vi "AI-DO-DAQ-OneShot.vi"(6 "Signal Generation":T1={"Signal Type"=enum."Sine Wave", "Amplitude"=1.0, "frequency"=10.0} {"frequency" format="%0.2p"; "Amplitude" format="%0.2p"}, 7 "Timing Parameters":cluster{"Rate":dbl, "Length (s)":dbl}={"Rate"=10000.0, "Length (s)"=1000.0} {"Rate" format="%0.2f"}, 8 "error in (no error)":errorcluster, 10 "Output":T2={"Physical Channel"="Dev2/ai1", "Minimum Value"=-10.0, "Maximum Value"=10.0} {"Maximum Value" format="%0.2f"; "Minimum Value" format="%0.2f"}, 11 "Input":T2={"Physical Channel"="Dev2/ai1", "Minimum Value"=-10.0, "Maximum Value"=10.0} {"Maximum Value" format="%0.2f"; "Minimum Value" format="%0.2f"}) -> (0 "error out":errorcluster, 2 "Rate":dbl=10000.0 caption="Actual Rate" format="%0.2f", 3 "Measurement":waveform(dbl)(graph))   [LabVIEW 2014]
doc: "I. Description:\nThis example demonstrates how to continuously acquire and generate data at the same time, synchronized with one another.\n\nII. Instructions for Running:\n1. Select the physical channel to correspond to where your signal is input on the DAQ device. Also, select the corresponding channel for where your signal is being generated.\n2. Enter the minimum and maximum voltage ranges.\nNote: For better accuracy try to match the input range to the expected voltage level of the measured signal.\n3. Set the Input/Output rate of the acquisition.\nNote: The rate should be at least twice as fast as the maximum frequency component of the signal being acquired. \n4. Select what type of signal to generate and the amplitude.\nNote: This example requires two DMA channels to run. If your hardware does not support two DMA channels, you need to set the Data Transfer Mechanism property for the Analog Output Task to use \"Interrupts\". The Data Transfer Mechanism property is located in the DAQmx Channel Property hierarchy at:\n\nDAQmx Channel Property Node>>Analog Output>>General Properties>>Advanced>>Data Transfer and Memory>>Data Transfer Mechanism\n\nRefer to your device documentation to determine how many DMA channels are supported for your hardware.\n\nIII. Block Diagram Steps:\n1. Create an analog input voltage channel. Also, create an analog output voltage channel.\n2. Set the rate for the sample clock. Additionally, define the sample mode to be continuous. Also, set the sample clock rate for the signal generation.\n2a. Call the Get Terminal Name with Device Prefix VI. This will take a Task and a terminal and create a properly formatted device + terminal name to use as the source of analog output.\n3. Find out what our actual Input/Output rate is \n4. Use the Basic Function Generator VI to create the signal to be generated.\n5. Call the Start VI to arm the two functions. Make sure the analog output is armed before the analog input. This will ensure both will start at the same time.\n6. Read the waveform data in a loop until the user hits the stop button or an error occurs. The Is Task Done? VI is used to check for errors in the Analog Output Task.\n7. Call the Clear VI to Clear the Task\n8. Use the popup dialog box to display an error if any.\n\nIV. I/O Connections Overview:\nMake sure your signal input/output terminals match the Physical Channel I/O controls."
uses:
  <vilib>/DAQmx/create/channels.llb/DAQmx Create Channel (AO-Voltage-Basic).vi
  <vilib>/DAQmx/configure/timing.llb/DAQmx Timing (Sample Clock).vi
  <vilib>/DAQmx/write.llb/DAQmx Write (Analog Wfm 1Chan NSamp).vi
  <vilib>/DAQmx/create/channels.llb/DAQmx Create Channel (AI-Voltage-Basic).vi
  <vilib>/DAQmx/read.llb/DAQmx Read (Analog Wfm 1Chan NSamp).vi
  <vilib>/measure/NI_MABase.lvlib
  <resource>/objmgr/daqmx.rc
panel:
  # "Channel Parameters"
  # "Timing Parameters"
  # "Signal Generation"
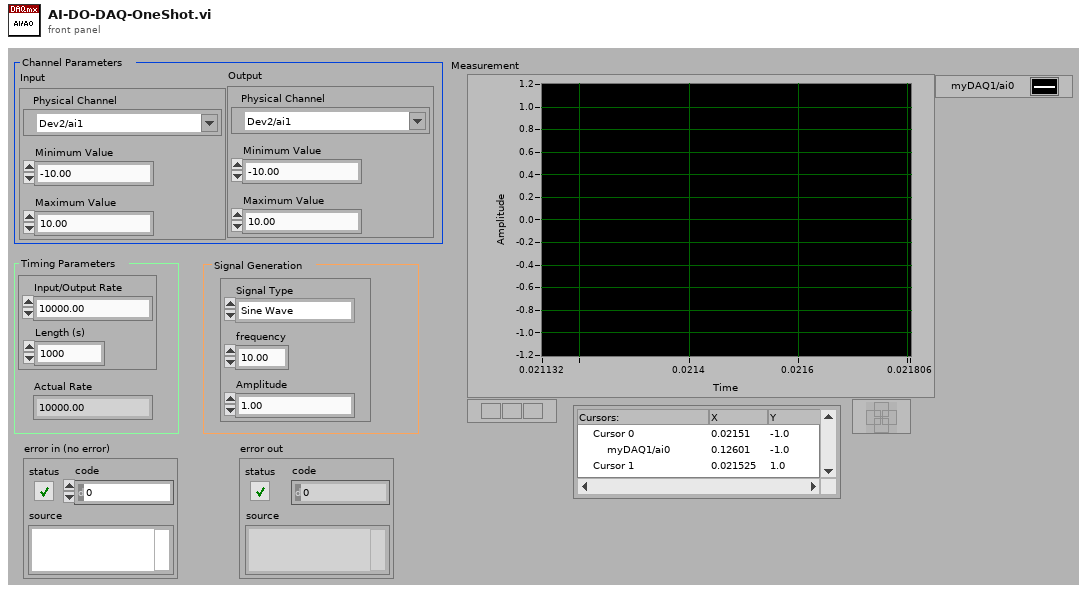
[diagram p1: front panel]
types:
  T1 = cluster{"Signal Type":enum16{"Sine Wave", "Triangle Wave", "Square Wave", "Sawtooth Wave"}, "Amplitude":dbl, "frequency":dbl}
  T2 = cluster{"Physical Channel":tag, "Minimum Value":dbl, "Maximum Value":dbl}
  T3 = enum16{"Sine Wave", "Triangle Wave", "Square Wave", "Sawtooth Wave"}
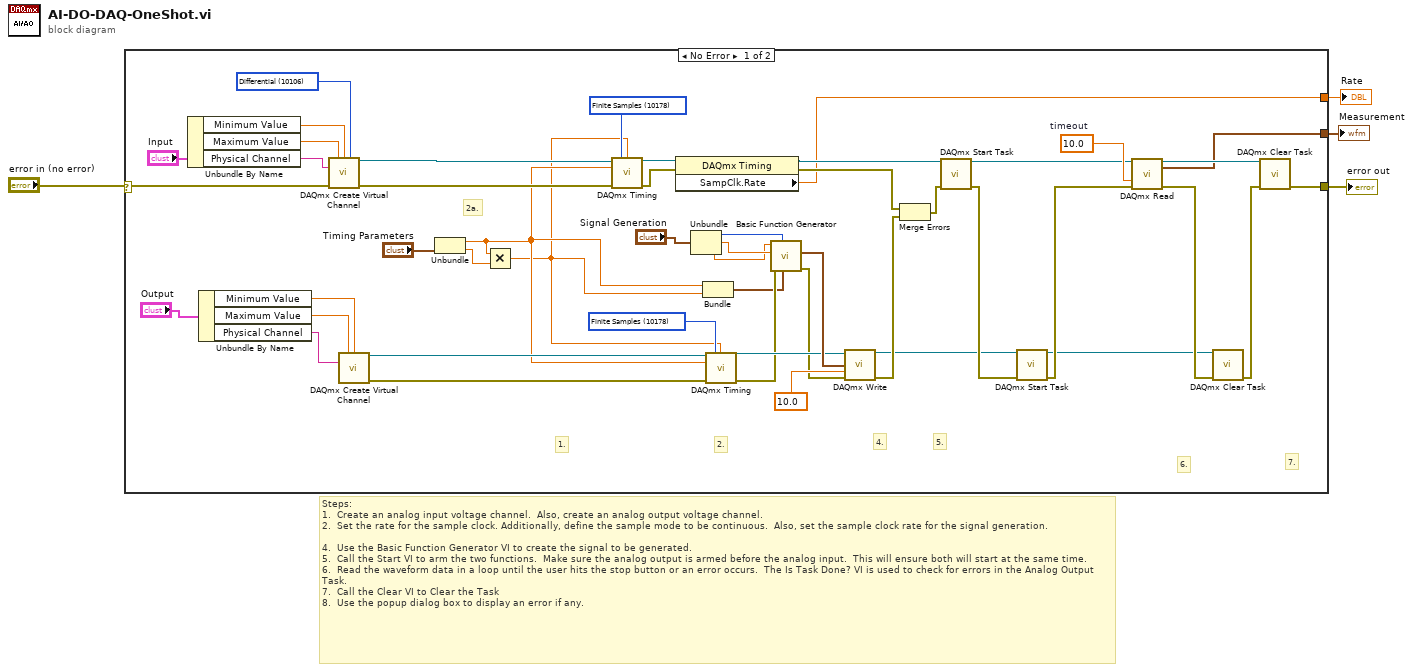
[diagram p0: block diagram]
diagram:
  # "Steps: \n1.  Create an analog input voltage channel.  Also, create an analog output voltage channel.\n2.  Set the rate for the sample clock. Additionally, define the sample mode to be continuous.  Also, set the sample clock rate for the signal generation.\n\n4.  Use the Basic Function Generator VI to create the signal to be generated.\n5.  Call the Start VI to arm the two functions.  Make sure the analog output is armed before the analog input.  This will ensure both will start at the same time.\n6.  Read the waveform data in a loop until the user hits the stop button or an error occurs.  The Is Task Done? VI is used to check for errors in the Analog Output Task.\n7.  Call the Clear VI to Clear the Task\n8.  Use the popup dialog box to display an error if any."
  n1 = case shown="No Error" "error in (no error)" {
    selector: "error in (no error)" -> [w10 w53]
    tunnel: [w44 w53] -> w3
    tunnel: [w9 _] -> w2
    tunnel: [w8 _] -> w1
    frame No Error {
      w31 = 10106 items=["default"=-1, "RSE"=10083, "NRSE"=10078, "Differential"=10106, "Pseudodifferential"=12529] ("input terminal configuration")
      w42 = 10.0  # timeout
      w50 = 10178 items=["Finite Samples"=10178, "Continuous Samples"=10123] ("sample mode")
      w51 = 10178 items=["Finite Samples"=10178, "Continuous Samples"=10123] ("sample mode")
      # "2a."
      # "6."
      # "4."
      # "5."
      # "7."
      # "2."
      # "1."
      n2 = Unbundle By Name("Input") -> ("Minimum Value"=w28:dbl, "Maximum Value"=w27:dbl, "Physical Channel"=w29:tag)
      n3 = Unbundle By Name("Output") -> ("Minimum Value"=w26:dbl, "Maximum Value"=w25:dbl, "Physical Channel"=w24:tag)
      n4 = call-poly <vilib>:"DAQmx Create Virtual Channel.vi"("maximum value"=w27, "minimum value"=w28, "input terminal configuration"=w31, "physical channels"=w29, "error in"=w10) -> ("task out"=w33:refnum<k21>, "error out"=w32:errorcluster)  [unwired: 9 in]
      n5 = call-poly <vilib>:"DAQmx Create Virtual Channel.vi"("maximum value"=w25, "minimum value"=w26, "physical channels"=w24) -> ("task out"=w49:refnum<k21>, "error out"=w48:errorcluster)  [unwired: 11 in]
      n6 = Unbundle("Timing Parameters") -> ("Rate"=w7:dbl, "Length (s)"=w11:dbl)
      n7 = Multiply(x=w7, y=w11) -> (x*y=w6:dbl)
      n8 = call-poly <vilib>:"DAQmx Timing.vi"("task/channels in"=w33, "sample mode"=w51, "samples per channel"=w6, "rate"=w7, "error in"=w32) -> ("task out"=w15:refnum<k21>, "error out"=w14:errorcluster)  [unwired: 9 in]
      n9 = property class="DAQmx Timing"(reference=w15, error in=w14) -> (reference out=w13:refnum<k21>, error out=w12:errorcluster, "SampClk.Rate"=w8:dbl)
      n10 = Unbundle("Signal Generation") -> ("Signal Type"=w21:T3, "Amplitude"=w20:dbl, "frequency"=w19:dbl)
      n11 = Bundle("Rate"=w7, w6) -> (w5:cluster{"Rate":dbl, dbl})  [unwired: 1 in]
      n12 = call-poly <vilib>:"DAQmx Timing.vi"("task/channels in"=w49, "sample mode"=w50, "samples per channel"=w6, "rate"=w7, "error in"=w48) -> ("task out"=w43:refnum<k21>, "error out"=w18:errorcluster)  [unwired: 9 in]
      n13 = call <vilib>:"Basic Function Generator.vi"("sampling info"=w5, "signal type"=w21, "error in (no error)"=w18, "amplitude"=w20, "frequency"=w19) -> ("error out"=w17:errorcluster, "signal out"=w46:waveform(dbl))  [unwired: 4 in, 1 out]
      n14 = call-poly <vilib>:"DAQmx Write.vi"("task/channels in"=w43, "data"=w46, "timeout"=10.0 ("Wirite Timeout"), "error in"=w17) -> ("task out"=w35:refnum<k21>, "error out"=w39:errorcluster)  [unwired: 9 in, 1 out]
      n15 = Merge Errors(w12, w39) -> (w38:errorcluster)
      n16 = call <vilib>:"DAQmx Start Task.vi"("task/channels in"=w13, "error in"=w38) -> ("task out"=w40:refnum<k21>, "error out"=w37:errorcluster)  [unwired: 12 in]
      n17 = call <vilib>:"DAQmx Start Task.vi"("task/channels in"=w35, "error in"=w37) -> ("task out"=w34:refnum<k21>, "error out"=w36:errorcluster)  [unwired: 12 in]
      n18 = call-poly <vilib>:"DAQmx Read.vi"("task/channels in"=w40, "timeout"=w42, "error in"=w36) -> ("task out"=w52:refnum<k21>, "data"=w9:waveform(dbl), "error out"=w41:errorcluster)  [unwired: 10 in]
      n19 = call <vilib>:"DAQmx Clear Task.vi"("task in"=w34, "error in"=w41) -> ("error out"=w45:errorcluster)  [unwired: 13 in]
      n20 = call <vilib>:"DAQmx Clear Task.vi"("task in"=w52, "error in"=w45) -> ("error out"=w44:errorcluster)  [unwired: 13 in]
    }
    frame Error {
    }
  }
  "error out" <- w3
  "Measurement" <- w2
  "Rate" <- w1
